vi "logical_series.create_logical_series.vi"(8 "error in":errorcluster, 10 "data":T1={"channel"="", "locator"={"type"="nominalLocator", "nominalLocator"={"channel"="", "tags"="", "type"=""}}, "dataSourceRid"=""}, 11 "Nominal Client in":refnum<class "Nominal Client.lvclass">) -> (0 "error out":errorcluster, 2 "Response":string, 3 "Nominal Client out":refnum<class "Nominal Client.lvclass">)   [LabVIEW 2018, in "Nominal Client.lvclass"]
doc: "Create a new logical series."
uses:
  Nominal Client.lvclass
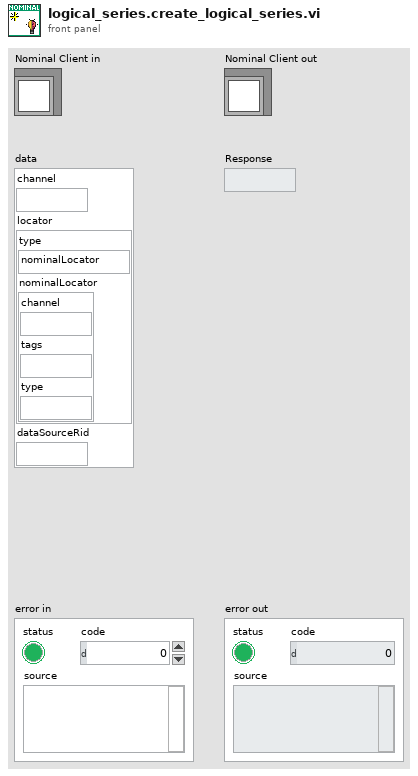
[diagram p1: front panel]
types:
  T1 = cluster{"channel":string, "locator":cluster{"type":string, "nominalLocator":cluster{"channel":string, "tags":string, "type":string}}, "dataSourceRid":string}
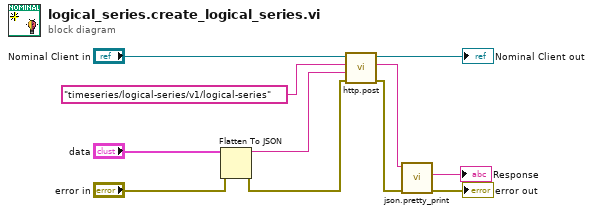
[diagram p0: block diagram]
diagram:
  n1 = Flatten To JSON(anything="data", error in (no error)="error in") -> (JSON string=w7:string, 11:w5:errorcluster)  [unwired: 1 in]
  n2 = call "http.post.vi"("error in"=w5, "Request body"=w7, "Path"="timeseries/logical-series/v1/logical-series", "Nominal Client in"="Nominal Client in") -> ("error out"=w1:errorcluster, "Response"=w4:string, "Nominal Client out"=→"Nominal Client out":refnum<class "Nominal Client.lvclass">)  [unwired: 4 in, 1 out]
  n3 = call "json.pretty_print.vi"("error in"=w1, "JSON in"=w4) -> ("error out"=→"error out":errorcluster, "Pretty JSON Out"=→"Response":string)  [unwired: 8 in]
